vi "Theta Align.vi"(5 "Time in flight":dbl=0.24969314401459508, 6 "Robot Velocities In":T2={"X Velocity"=-0.0, "Y Velocity"=0.0, "Rotational \nVelocity"=-0.0}) -> (2 "Robot Velocities Out":T2={"X Velocity"=-0.0, "Y Velocity"=0.0, "Rotational \nVelocity"=5.043625671549705})   [LabVIEW 2025]
uses:
  swerve-template/Type Definitions/Data/Robot Velocities.ctl
  <vilib>/Rock Robotics/Network Tables/NT Read Number.vi
  Framework/Robot Global Data.vi
  <vilib>/addons/control/pid/pid.llb/PID (DBL).vi
  <vilib>/addons/control/pid/NI_PID_pid.lvlib
panel:
  in  "F term":dbl=8.0
  in  "Test angle":dbl=-60.0
  in  "Test with given angle":bool
  out "Pid tuner":cluster{"upper limit":dbl, "upper limit":dbl}(graph)={"upper limit"=-38.44536774908863, "upper limit"=-36.42791748046875}
  in  "output range":cluster{"output high":dbl, "output low":dbl}={"output high"=700.0, "output low"=-700.0} {"output low" format="%.2f"; "output high" format="%.2f"}
  in  "PID gains":T1={"proportional gain (Kc)"=2.5, "integral time (Ti, min)"=0.0, "derivative time (Td, min)"=0.0} {"derivative time (Td, min)" format="%.3f"; "integral time (Ti, min)" format="%.3f"; "proportional gain (Kc)" format="%.3f"}
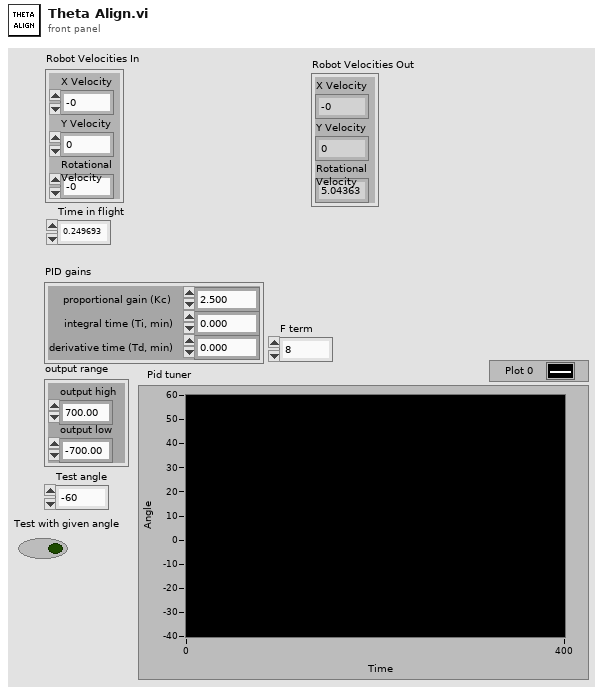
[diagram p1: front panel]
types:
  T1 = cluster{"proportional gain (Kc)":dbl, "integral time (Ti, min)":dbl, "derivative time (Td, min)":dbl}
  T2 = typedef "Robot Velocities.ctl" = cluster{"X Velocity":dbl, "Y Velocity":dbl, "Rotational \nVelocity":dbl}
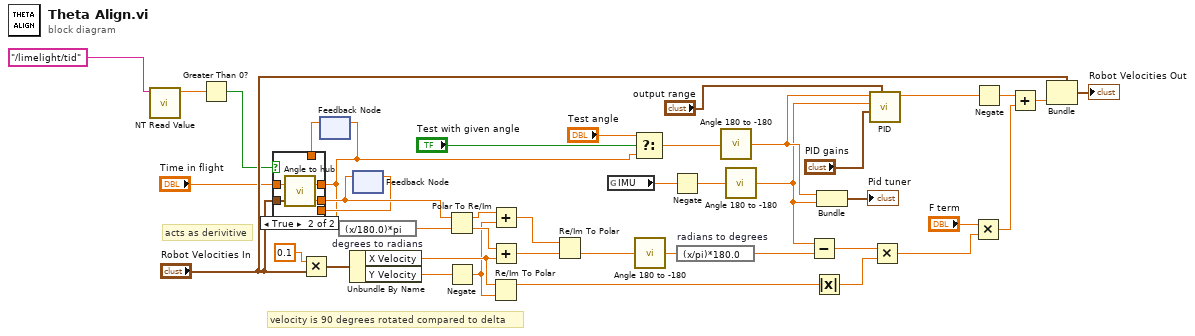
[diagram p0: block diagram]
diagram:
  # "acts as derivitive"
  # "velocity is 90 degrees rotated compared to delta"
  n1 = call-poly <vilib>:"NT Read Value.vi"("name"="/limelight/tid") -> ("value"=w6:dbl)  [unwired: 8 in, 2 out]
  n2 = Greater Than 0?(x=w6) -> (x > 0?=w5:bool)
  n3 = Multiply(x=0.1, y="Robot Velocities In") -> (x*y=w34:T2)
  n4 = feedback #1() -> (w4:dbl)  [unwired: 1 in]
  n5 = Unbundle By Name(w34) -> ("X Velocity"=w19:dbl, "Y Velocity"=w16:dbl)
  n6 = feedback #2() -> (w2:dbl)  [unwired: 1 in]
  n7 = case shown="True" w5 {
    tunnel: [w43 w48] -> w3
    tunnel: [w44 w47] -> w1
    tunnel: "Robot Velocities In" -> [_ w46]
    tunnel: "Time in flight" -> [_ w45]
    tunnel: w4 -> [w44 _]
    tunnel: w2 -> [w43 _]
    frame False {
    }
    frame True {
      n8 = call "Angle to hub.vi"("Robot Velocities In"=w46, "Time in flight"=w45) -> ("Distance to hub"=w48:dbl, "Angle to hub"=w47:dbl)
    }
  }
  n9 = feedback-in #1(w1) -> ()
  n10 = expression code="(x/180.0)*pi" "degrees to radians"(w1) -> (w26:dbl)
  n11 = feedback-in #2(w3) -> ()
  n12 = Polar To Re/Im(2:w26, 3:w3) -> (0:w25:dbl, 1:w18:dbl)
  n13 = Negate(x=w16) -> (-x=w15:dbl)
  n14 = Add(x=w18, y=w15) -> (x+y=w17:dbl)
  n15 = Add(x=w25, y=w19) -> (x+y=w24:dbl)
  n16 = Re/Im To Polar(2:w15, 3:w19) -> (1:w20:dbl)  [unwired: 1 out]
  n17 = Re/Im To Polar(2:w24, 3:w17) -> (0:w14:dbl)  [unwired: 1 out]
  n18 = global read "Robot Global Data.vi" "IMU"() -> (w9:dbl)
  n19 = Select(t="Test angle", s="Test with given angle", f=w1) -> (s? t:f=w36:dbl)
  n20 = call "Angle 180 to -180.vi"("Angle in"=w14) -> ("Angle out"=w13:dbl)
  n21 = Negate(x=w9) -> (-x=w8:dbl)
  n22 = expression code="(x/pi)*180.0" "radians to degrees"(w13) -> (w23:dbl)
  n23 = call "Angle 180 to -180.vi"("Angle in"=w36) -> ("Angle out"=w35:dbl)
  n24 = call "Angle 180 to -180.vi"("Angle in"=w8) -> ("Angle out"=w12:dbl)
  n25 = Subtract(x=w12, y=w23) -> (x-y=w32:dbl)
  n26 = Absolute Value(x=w20) -> (abs(x)=w27:dbl)
  n27 = Bundle("Angle out"=w35, "Angle out"=w12) -> (→"Pid tuner":cluster{"Angle out":dbl, "Angle out":dbl})  [unwired: 1 in]
  n28 = call-poly <vilib>:"PID.vi"("output range"="output range", "PID gains"="PID gains", "process variable"=w12, "setpoint"=w35) -> ("output"=w28:dbl)  [unwired: 6 in, 1 out]
  n29 = Multiply(x=w32, y=w27) -> (x*y=w31:dbl)
  n30 = Multiply(x="F term", y=w31) -> (x*y=w29:dbl)
  n31 = Negate(x=w28) -> (-x=w21:dbl)
  n32 = Add(x=w21, y=w29) -> (x+y=w22:dbl)
  n33 = Bundle(cluster="Robot Velocities In", "Rotational \nVelocity"=w22) -> (→"Robot Velocities Out":T2)  [unwired: 2 in]
